vi "local.Get Generic Property (Core).vi"(0 "SLSC Local in":refnum<class "SLSC Interface.lvclass">, 1 "property type":T1, 5 "resources":string, 7 "property":refnum<k21>, 11 "error in (no error)":errorcluster) -> (4 "SLSC Local out":refnum<class "SLSC Interface.lvclass">, 10 "property value":variant, 15 "error out":errorcluster)   [LabVIEW 2016, in "SLSC Interface.lvclass"]
uses:
  SLSC Interface Class/SLSC Interface.lvclass
  SLSC Interface Class/Property Type.ctl
  SLSC Interface Class/Read session.vi
  <vilib>/SLSC/Get Generic Property (Bool).vi
  <vilib>/SLSC/Get Generic Property (DBL).vi
  <vilib>/SLSC/Get Generic Property (I32).vi
  <vilib>/SLSC/Get Generic Property (I64).vi
  <vilib>/SLSC/Get Generic Property (String).vi
  <vilib>/SLSC/Get Generic Property (U32).vi
  <vilib>/SLSC/Get Generic Property (U64).vi
  <vilib>/SLSC/Get Generic Property (1D Bool).vi
  <vilib>/SLSC/Get Generic Property (1D DBL).vi
  <vilib>/SLSC/Get Generic Property (1D I32).vi
  <vilib>/SLSC/Get Generic Property (1D I64).vi
  <vilib>/SLSC/Get Generic Property (1D String).vi
  <vilib>/SLSC/Get Generic Property (1D U32).vi
  <vilib>/SLSC/Get Generic Property (1D U64).vi
  SLSC Interface Class/Write session.vi
  <vilib>/SLSC/SLSC.lvlib
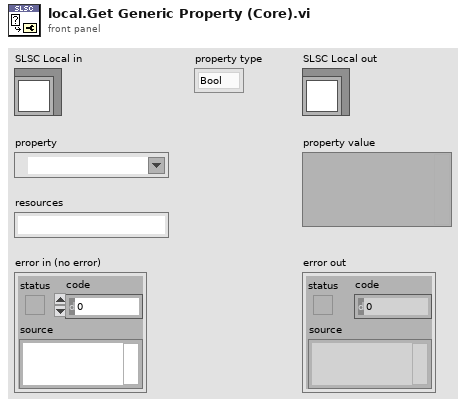
[diagram p1: front panel]
types:
  T1 = typedef "SLSC Interface.lvclass/Property Type.ctl" = enum16{"Bool", "DBL", "I32", "I64", "String", "U32", "U64", "1D Bool", "1D DBL", "1D I32", "1D I64", "1D String", "1D U32", "1D U64"}
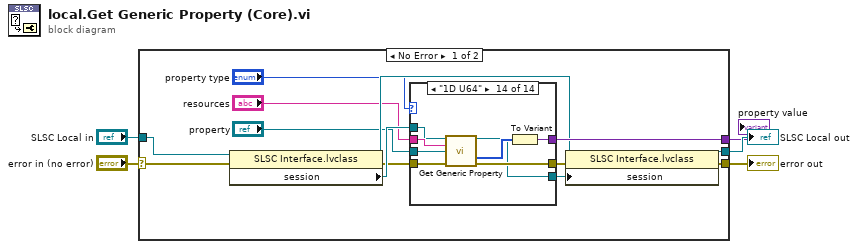
[diagram p0: block diagram]
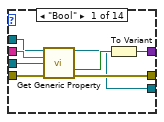
[diagram p2: hidden frame]
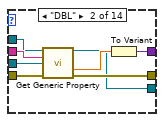
[diagram p3: hidden frame]
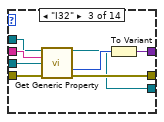
[diagram p4: hidden frame]
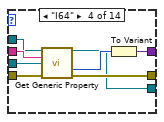
[diagram p5: hidden frame]
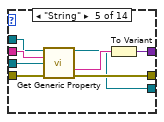
[diagram p6: hidden frame]
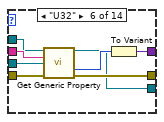
[diagram p7: hidden frame]
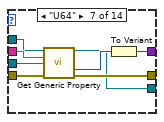
[diagram p8: hidden frame]
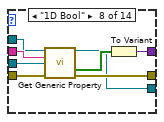
[diagram p9: hidden frame]
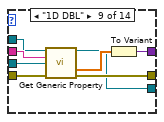
[diagram p10: hidden frame]
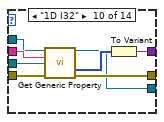
[diagram p11: hidden frame]
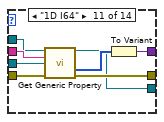
[diagram p12: hidden frame]
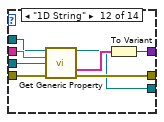
[diagram p13: hidden frame]
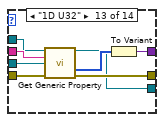
[diagram p14: hidden frame]
diagram:
  n1 = case shown="No Error" "error in (no error)" {
    selector: "error in (no error)" -> [w12 w132]
    tunnel: [w9 w132] -> w4
    tunnel: [w15 w131] -> w2
    tunnel: "SLSC Local in" -> [w17 w131]
    tunnel: [w18 _] -> w1
    frame No Error {
      n2 = property class="SLSC Interface.lvclass"(reference=w17, error in=w12) -> (reference out=w16:refnum<class "SLSC Interface.lvclass">, error out=w11:errorcluster, "session"=w14:refnum<k21>)
      n3 = case shown="\"1D U64\"" "property type" {
        tunnel: "resources" -> [w26 w34 w42 w50 w58 w66 w74 w82 w90 w98 w106 w114 w122 w130]
        tunnel: "property" -> [w25 w33 w41 w49 w57 w65 w73 w81 w89 w97 w105 w113 w121 w129]
        tunnel: [w23 w31 w39 w47 w55 w63 w71 w79 w87 w95 w103 w111 w119 w127] -> w18
        tunnel: w11 -> [w22 w30 w38 w46 w54 w62 w70 w78 w86 w94 w102 w110 w118 w126]
        tunnel: [w21 w29 w37 w45 w53 w61 w69 w77 w85 w93 w101 w109 w117 w125] -> w10
        tunnel: w14 -> [w20 w28 w36 w44 w52 w60 w68 w76 w84 w92 w100 w108 w116 w124]
        tunnel: [w19 w27 w35 w43 w51 w59 w67 w75 w83 w91 w99 w107 w115 w123] -> w13
        frame "Bool" {
          n4 = call-poly <vilib>:"Get Generic Property.vi"("session in"=w20, "resources"=w26, "property"=w25, "error in (no error)"=w22) -> ("session out"=w19:refnum<k21>, "property value"=w24:bool, "error out"=w21:errorcluster)  [unwired: 9 in]
          n5 = To Variant(anything=w24) -> (Variant=w23:variant)
        }
        frame "DBL" {
          n6 = call-poly <vilib>:"Get Generic Property.vi"("session in"=w28, "resources"=w34, "property"=w33, "error in (no error)"=w30) -> ("session out"=w27:refnum<k21>, "property value"=w32:dbl, "error out"=w29:errorcluster)  [unwired: 9 in]
          n7 = To Variant(anything=w32) -> (Variant=w31:variant)
        }
        frame "I32" {
          n8 = call-poly <vilib>:"Get Generic Property.vi"("session in"=w36, "resources"=w42, "property"=w41, "error in (no error)"=w38) -> ("session out"=w35:refnum<k21>, "property value"=w40:i32, "error out"=w37:errorcluster)  [unwired: 9 in]
          n9 = To Variant(anything=w40) -> (Variant=w39:variant)
        }
        frame "I64" {
          n10 = call-poly <vilib>:"Get Generic Property.vi"("session in"=w44, "resources"=w50, "property"=w49, "error in (no error)"=w46) -> ("session out"=w43:refnum<k21>, "property value"=w48:i64, "error out"=w45:errorcluster)  [unwired: 9 in]
          n11 = To Variant(anything=w48) -> (Variant=w47:variant)
        }
        frame "String" {
          n12 = call-poly <vilib>:"Get Generic Property.vi"("session in"=w52, "resources"=w58, "property"=w57, "error in (no error)"=w54) -> ("session out"=w51:refnum<k21>, "property value"=w56:string, "error out"=w53:errorcluster)  [unwired: 9 in]
          n13 = To Variant(anything=w56) -> (Variant=w55:variant)
        }
        frame "U32" {
          n14 = call-poly <vilib>:"Get Generic Property.vi"("session in"=w60, "resources"=w66, "property"=w65, "error in (no error)"=w62) -> ("session out"=w59:refnum<k21>, "property value"=w64:u32, "error out"=w61:errorcluster)  [unwired: 9 in]
          n15 = To Variant(anything=w64) -> (Variant=w63:variant)
        }
        frame "U64" {
          n16 = call-poly <vilib>:"Get Generic Property.vi"("session in"=w68, "resources"=w74, "property"=w73, "error in (no error)"=w70) -> ("session out"=w67:refnum<k21>, "property value"=w72:u64, "error out"=w69:errorcluster)  [unwired: 9 in]
          n17 = To Variant(anything=w72) -> (Variant=w71:variant)
        }
        frame "1D Bool" {
          n18 = call-poly <vilib>:"Get Generic Property.vi"("session in"=w76, "resources"=w82, "property"=w81, "error in (no error)"=w78) -> ("session out"=w75:refnum<k21>, "property value"=w80:bool[], "error out"=w77:errorcluster)  [unwired: 9 in]
          n19 = To Variant(anything=w80) -> (Variant=w79:variant)
        }
        frame "1D DBL" {
          n20 = call-poly <vilib>:"Get Generic Property.vi"("session in"=w84, "resources"=w90, "property"=w89, "error in (no error)"=w86) -> ("session out"=w83:refnum<k21>, "property value"=w88:dbl[], "error out"=w85:errorcluster)  [unwired: 9 in]
          n21 = To Variant(anything=w88) -> (Variant=w87:variant)
        }
        frame "1D I32" {
          n22 = call-poly <vilib>:"Get Generic Property.vi"("session in"=w92, "resources"=w98, "property"=w97, "error in (no error)"=w94) -> ("session out"=w91:refnum<k21>, "property value"=w96:i32[], "error out"=w93:errorcluster)  [unwired: 9 in]
          n23 = To Variant(anything=w96) -> (Variant=w95:variant)
        }
        frame "1D I64" {
          n24 = call-poly <vilib>:"Get Generic Property.vi"("session in"=w100, "resources"=w106, "property"=w105, "error in (no error)"=w102) -> ("session out"=w99:refnum<k21>, "property value"=w104:i64[], "error out"=w101:errorcluster)  [unwired: 9 in]
          n25 = To Variant(anything=w104) -> (Variant=w103:variant)
        }
        frame "1D String" {
          n26 = call-poly <vilib>:"Get Generic Property.vi"("session in"=w108, "resources"=w114, "property"=w113, "error in (no error)"=w110) -> ("session out"=w107:refnum<k21>, "property value"=w112:string[], "error out"=w109:errorcluster)  [unwired: 9 in]
          n27 = To Variant(anything=w112) -> (Variant=w111:variant)
        }
        frame "1D U32" {
          n28 = call-poly <vilib>:"Get Generic Property.vi"("session in"=w116, "resources"=w122, "property"=w121, "error in (no error)"=w118) -> ("session out"=w115:refnum<k21>, "property value"=w120:u32[], "error out"=w117:errorcluster)  [unwired: 9 in]
          n29 = To Variant(anything=w120) -> (Variant=w119:variant)
        }
        frame "1D U64" {
          n30 = call-poly <vilib>:"Get Generic Property.vi"("session in"=w124, "resources"=w130, "property"=w129, "error in (no error)"=w126) -> ("session out"=w123:refnum<k21>, "property value"=w128:u64[], "error out"=w125:errorcluster)  [unwired: 9 in]
          n31 = To Variant(anything=w128) -> (Variant=w127:variant)
        }
      }
      n32 = property class="SLSC Interface.lvclass"(reference=w16, error in=w10, "session"=w13) -> (reference out=w15:refnum<class "SLSC Interface.lvclass">, error out=w9:errorcluster)
    }
    frame Error {
    }
  }
  "error out" <- w4
  "SLSC Local out" <- w2
  "property value" <- w1
